vi "Versioned Load.vi"(5 "path":path) -> (1 "Overall":cluster{"Time (s)":dbl, "Distance (ft)":dbl}, 3 "Points out":cluster{"x":dbl, "y":dbl, "th":dbl}[](array[cluster]), 4 "Commands out":cluster{"Time (s)":dbl, T8, bool}[](array[cluster]), 6 "Zero V":bool, 8 "Reversals":T10, 10 "Trajectory Data":T1, 12 "Trajectory Meta":cluster{"Drive Type":T3, "Path Type":T4}, 14 "Fields":T7 {"Overrides"."Angle Override" step=5.0; "Overrides"."Velocity Override" step=5.0; "Overrides"."Angular Override" step=5.0; "Angular Limits"."Jerk (deg/s^3)" min=0.0 step=1.0; "Angular Limits"."Accel (deg/s^2)" min=0.0; "Angular Limits"."Velocity (deg/s)" min=0.0}, 15 "Auto Align":bool)   [LabVIEW 2025]
uses:
  Types/Single Cmd Info.ctl
  <vilib>/picture/picture.llb/imagedata.ctl
  Types/Overrides.ctl
  Types/Angluar Limits.ctl
  Types/Drive Type.ctl
  Types/Path Type.ctl
  Types/Trajectory Data.ctl
  Types/Segment Type.ctl
  Types/Availible Command systems for auto.ctl
  Types/Limits.ctl
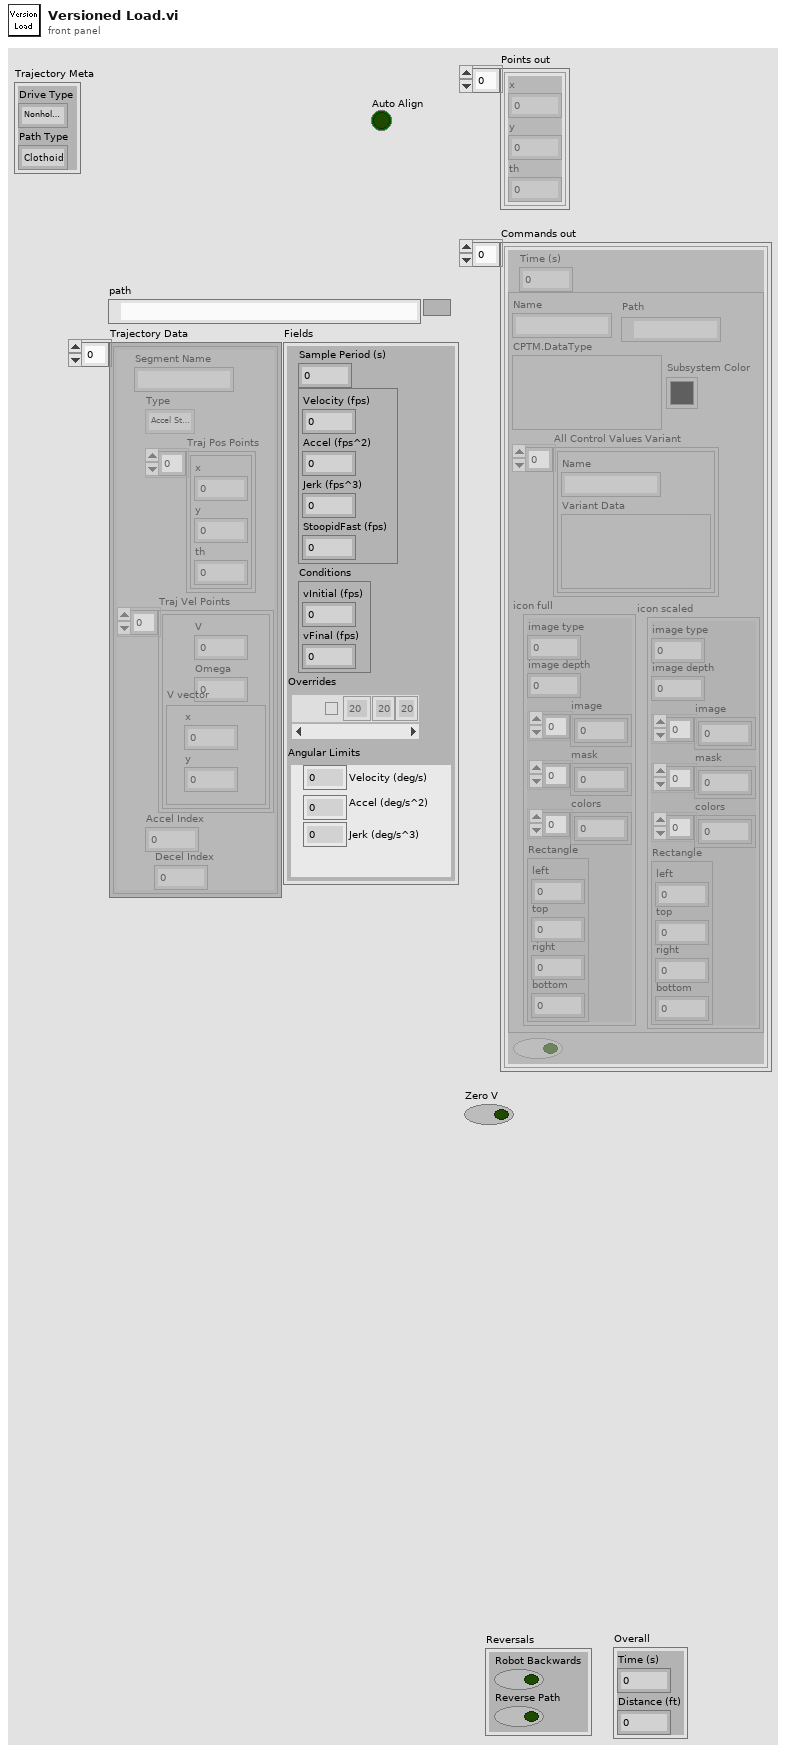
[diagram p1: front panel]
types:
  T1 = typedef "Trajectory Data.ctl" = cluster{"Segment Name":string, "Type":T2, "Traj Pos Points":cluster{"x":dbl, "y":dbl, "th":dbl}[], "Traj Vel Points":cluster{"V":dbl, "Omega":dbl, "V vector":cluster{"y":dbl, "x":dbl}}[], "Accel Index":i32, "Decel Index":i32}[]
  T2 = typedef "Segment Type.ctl" = enum16{"Accel Straight", "Const Straight", "Blend", "Circle", "Bezier"}
  T3 = typedef "Drive Type.ctl" = enum16{"Nonholonomic", "Holonomic"}
  T4 = typedef "Path Type.ctl" = enum16{"Clothoid", "Bezier"}
  T5 = typedef "Overrides.ctl" = cluster{"Count":string, "Angular Override":dbl, "Enabled?":bool, "Velocity Override":dbl, "Angle Override":dbl}[]
  T6 = typedef "Angluar Limits.ctl" = cluster{"Velocity (deg/s)":dbl, "Accel (deg/s^2)":dbl, "Jerk (deg/s^3)":dbl}
  T7 = cluster{"Sample Period (s)":dbl, cluster{"Velocity (fps)":dbl, "Accel (fps^2)":dbl, "Jerk (fps^3)":dbl, "StoopidFast (fps)":dbl}, "Conditions":cluster{"vInitial (fps)":dbl, "vFinal (fps)":dbl}, "Overrides":T5, "Angular Limits":T6}
  T8 = typedef "Single Cmd Info.ctl" = cluster{"Name":string, "CPTM.DataType":variant, "All Control Values Variant":cluster{"Name":string, "Variant Data":variant}[], "icon full":T9, "icon scaled":T9, "Path":path, "Subsystem Color":u32}
  T9 = typedef "imagedata.ctl" = cluster{"image type":i32, "image depth":i32, "image":u8[], "mask":u8[], "colors":u32[], "Rectangle":cluster{"left":i16, "top":i16, "right":i16, "bottom":i16}}
  T10 = cluster{"Robot Backwards":bool, "Reverse Path":bool}
  T11 = cluster{"Segment Name":string, "Type":T2, "Traj Pos Points":cluster{"x":dbl, "y":dbl, "th":dbl}[], "Traj Vel Points":cluster{"V":dbl, "Omega":dbl}[], "Accel Index":i32, "Decel Index":i32}[]
  T12 = cluster{"Sample Period (s)":dbl, "Limits 2":cluster{"Velocity (fps)":dbl, "Acceleration (fps^2)":dbl, "Jerk (fps^3)":dbl}, "Conditions":cluster{"vInitial (fps)":dbl, "vFinal (fps)":dbl}, " Acceleration Overrides":cluster{"Angular \nAccelerations":dbl[], "Accel Override Bools":bool[]}}
  T13 = cluster{"Velocity":dbl, "Sample Time":dbl, "Accel":dbl}
  T14 = cluster{"Sample Period (s)":dbl, "Limits":cluster{"Velocity (fps)":dbl, "Acceleration (fps^2)":dbl, "Jerk (fps^3)":dbl}, "Conditions":cluster{"vInitial (fps)":dbl, "vFinal (fps)":dbl}}
  T15 = cluster{"Sample Period (s)":dbl, "Limits":cluster{"Velocity (fps)":dbl, "Acceleration (fps^2)":dbl, "Jerk (fps^3)":dbl}, "Conditions":cluster{"vInitial (fps)":dbl, "vFinal (fps)":dbl}, "Min Rads":dbl[]}
  T16 = typedef "Availible Command systems for auto.ctl" = u16
  T17 = cluster{"Time into Path":dbl, "System":T16, "Item Selected?":bool, "System Selection":T16}[]
  T18 = cluster{"Sample Period (s)":dbl, "Limits 2":cluster{"Velocity (fps)":dbl, "Acceleration (fps^2)":dbl, "Jerk (fps^3)":dbl, "Stoopid Fast":dbl}, "Conditions":cluster{"vInitial (fps)":dbl, "vFinal (fps)":dbl}, " Acceleration Overrides":cluster{"Angular \nAccelerations":dbl[], "Accel Override Bools":bool[]}}
  T19 = cluster{"Sample Period (s)":dbl, "Limits":cluster{"Velocity (fps)":dbl, "Accel (fps^2)":dbl, "Turn Accel (fps^2)":dbl, "Jerk (fps^3)":dbl}, "Conditions":cluster{"vInitial (fps)":dbl, "vFinal (fps)":dbl}, cluster{dbl[], bool[]}}
  T20 = cluster{"Reverse Path":bool, "Robot Backwards":bool}
  T21 = typedef "Limits.ctl" = cluster{"Velocity (fps)":dbl, "Accel (fps^2)":dbl, "Jerk (fps^3)":dbl, "StoopidFast (fps)":dbl}
  T22 = cluster{"Sample Period (s)":dbl, "Limits":T21, "Conditions":cluster{"vInitial (fps)":dbl, "vFinal (fps)":dbl}, "Overrides":T5, "Angular Limits":T6}
  T23 = cluster{"Velocity":dbl, "Accel":dbl, "Accel":dbl, "Velocity":dbl}
  T24 = cluster{"Velocity (fps)":dbl, "Acceleration (fps^2)":dbl, "Jerk (fps^3)":dbl}
  T25 = cluster{"vInitial (fps)":dbl, "vFinal (fps)":dbl}
  T26 = cluster{"Velocity (fps)":dbl, "Acceleration (fps^2)":dbl, "Jerk (fps^3)":dbl, "Velocity (fps)":dbl}
  T27 = cluster{string, "Angular Multiplier":dbl, bool, "Velocity (fps)":dbl, "Velocity (fps)":dbl}
  T28 = cluster{"Angular \nAccelerations":dbl[], "Accel Override Bools":bool[]}
  T29 = cluster{"Velocity (fps)":dbl, "Acceleration (fps^2)":dbl, "Jerk (fps^3)":dbl, "Stoopid Fast":dbl}
  T30 = cluster{"Velocity (fps)":dbl, "Accel (fps^2)":dbl, "Turn Accel (fps^2)":dbl, "Jerk (fps^3)":dbl}
  T31 = cluster{"Velocity (fps)":dbl, "Accel (fps^2)":dbl, "Jerk (fps^3)":dbl, "StoopidFast (fps)":dbl}
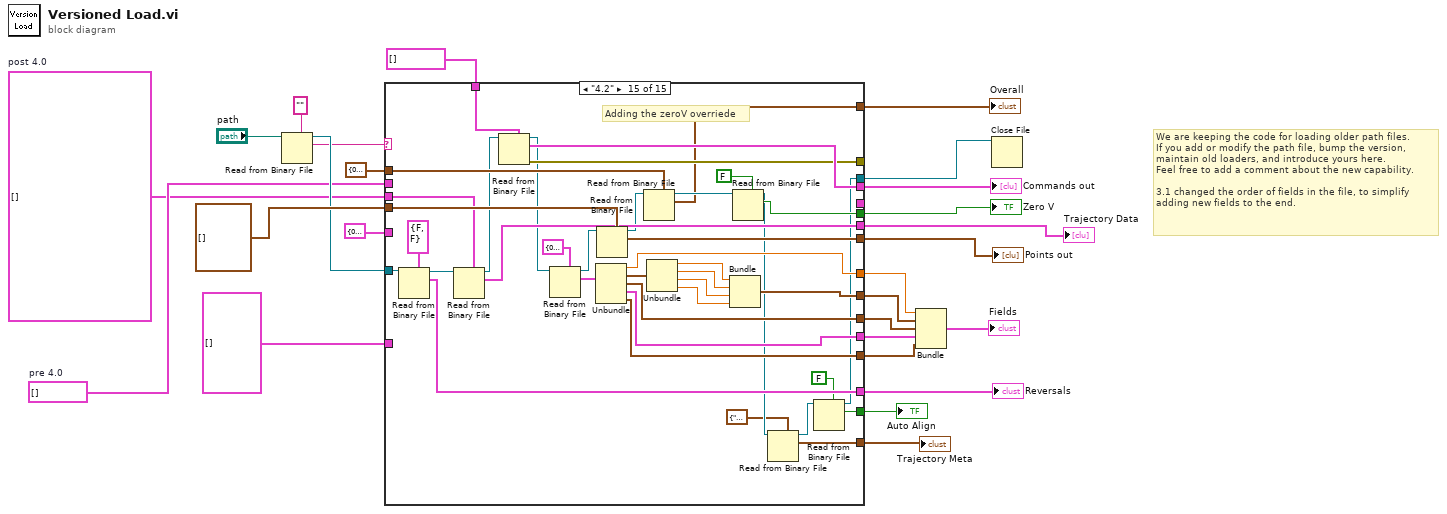
[diagram p0: block diagram]
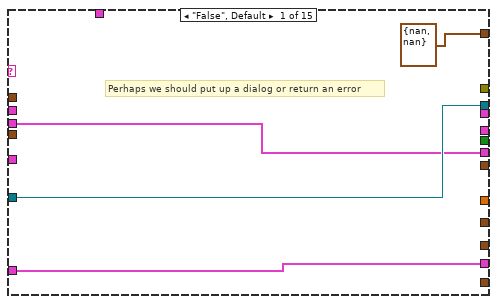
[diagram p2: hidden frame]
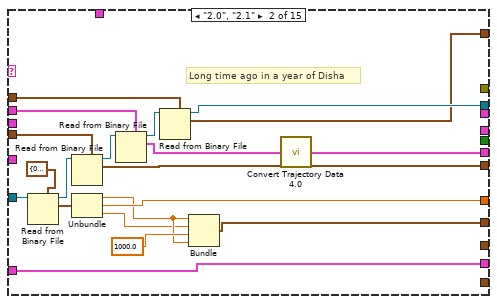
[diagram p3: hidden frame]
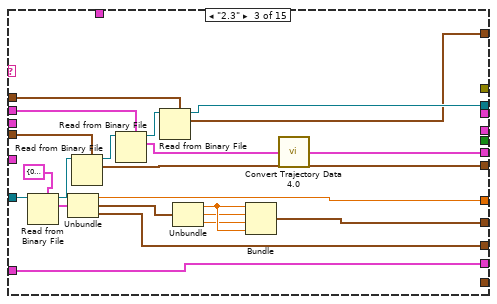
[diagram p4: hidden frame]
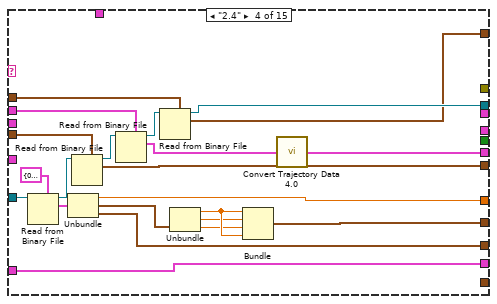
[diagram p5: hidden frame]
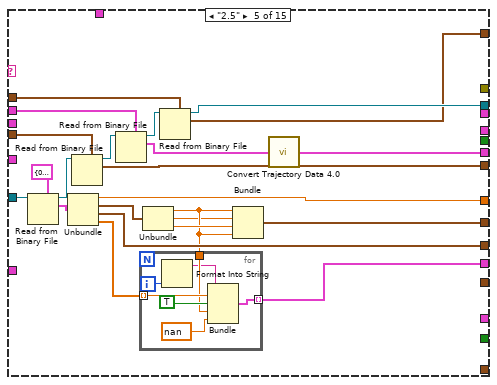
[diagram p6: hidden frame]
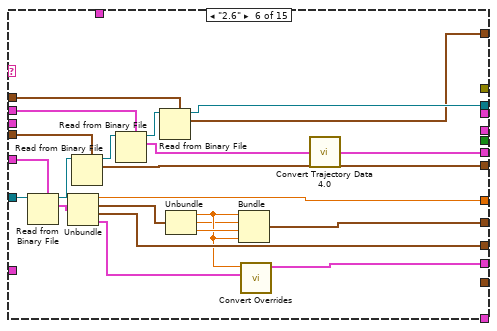
[diagram p7: hidden frame]
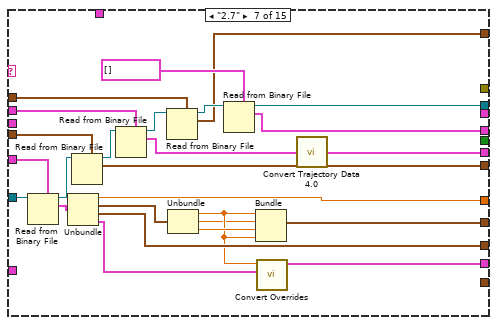
[diagram p8: hidden frame]
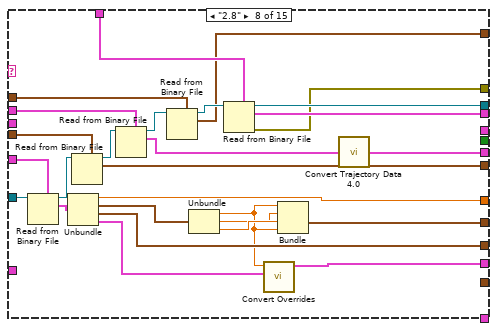
[diagram p9: hidden frame]
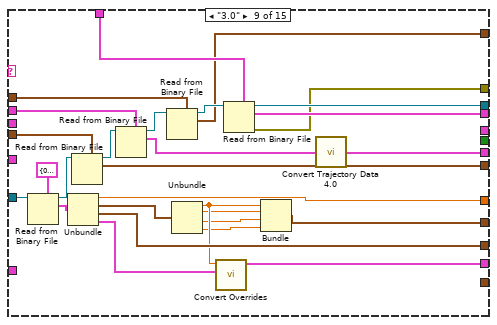
[diagram p10: hidden frame]
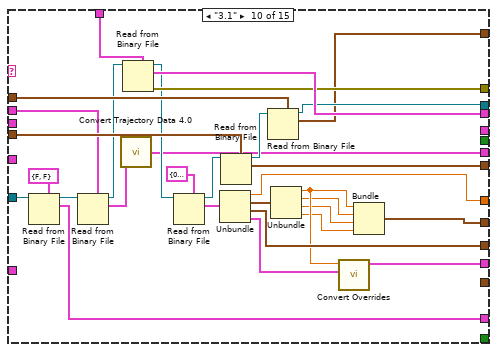
[diagram p11: hidden frame]
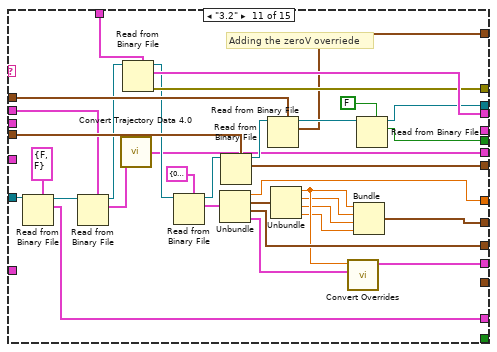
[diagram p12: hidden frame]
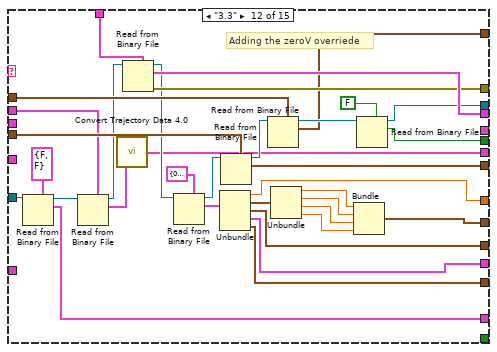
[diagram p13: hidden frame]
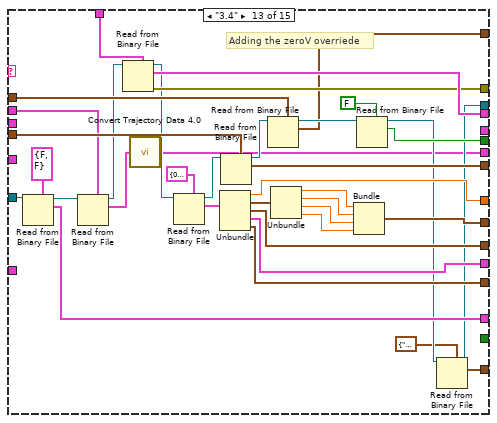
[diagram p14: hidden frame]
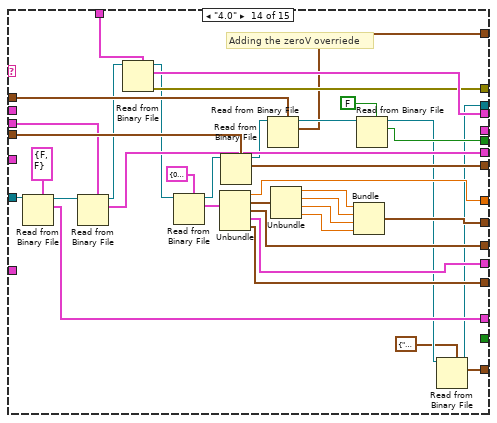
[diagram p15: hidden frame]
diagram:
  w4 = T11 []  # pre 4.0
  w3 = T1 []  # post 4.0
  # "We are keeping the code for loading older path files.\nIf you add or modify the path file, bump the version,\nmaintain old loaders, and introduce yours here.\nFeel free to add a comment about the new capability.\n\n3.1 changed the order of fields in the file, to simplify\nadding new fields to the end."
  n1 = Read from Binary File(5:"" ("String"), 11:"path") -> (2:w10:string, 3:w11:refnum<file>)  [unwired: 4 in, 2 out]
  n2 = case shown="\"4.2\"" w10 {
    tunnel: w11 -> [w30 w49 w71 w93 w116 w146 w172 w199 w227 w248 w282 w316 w353 w390 w429]
    tunnel: cluster{"x":dbl, "y":dbl, "th":dbl}[] [] ("Points in") -> [_ w47 w69 w91 w114 w144 w170 w197 w225 w257 w291 w325 w362 w398 w437]
    tunnel: [_ w46 w68 w90 w113 w143 w169 w196 w224 w256 w290 w324 w361 w397 w436] -> w16
    tunnel: w4 -> [_ w45 w67 w89 w112 w142 w168 w195 w223 w255 w289 w323 w360 _ _]
    tunnel: cluster{"Time (s)":dbl, "Distance (ft)":dbl} {"Time (s)"=0.0, "Distance (ft)"=0.0} ("Cluster 4") -> [_ w43 w65 w87 w110 w140 w166 w193 w221 w254 w288 w322 w359 w396 w435]
    tunnel: [w30 w41 w63 w85 w108 w138 w160 w187 w215 w244 w264 w301 w330 w367 w403] -> w13
    tunnel: [_ w39 w62 w84 w107 w137 w164 w191 w219 w231 w266 w303 w340 w377 w416] -> w23
    tunnel: [_ w35 w56 w77 w101 w132 w154 w182 w203 w236 w271 w308 w345 w382 w421] -> w24
    tunnel: [_ _ w61 w83 w106 w136 w163 w190 w218 w253 w287 w321 w358 w395 w434] -> w25
    tunnel: [w29 w34 w55 w76 w100 w130 w151 w179 w209 w240 w275 w296 w334 w371 w410] -> w26
    tunnel: [w27 w31 w51 w73 w95 w125 w148 w174 w201 w229 w260 w294 w328 w394 w433] -> w2
    tunnel: [_ _ _ _ _ _ w159 _ _ _ _ _ _ _ _] -> _
    tunnel: cluster{"Time (s)":dbl, T8, bool}[] [] ("Commands in") -> [_ _ _ _ _ _ _ w186 w214 w251 w285 w319 w356 w393 w432]
    tunnel: [_ _ _ _ _ _ _ w185 w213 w250 w284 w318 w355 w392 w431] -> w18
    tunnel: [_ _ _ _ _ _ _ w184 w212 w249 w283 w317 w354 w391 w430] -> _
    tunnel: T12 {"Sample Period (s)"=0.0, "Limits 2"={"Velocity (fps)"=0.0, "Acceleration (fps^2)"=0.0, "Jerk (fps^3)"=0.0}, "Conditions"={"vInitial (fps)"=0.0, "vFinal (fps)"=0.0}, " Acceleration Overrides"={"Angular \nAccelerations"=[], "Accel Override Bools"=[]}} ("Cluster") -> [_ _ _ _ _ w134 w157 w180 _ _ _ _ _ _ _]
    tunnel: [_ _ _ _ _ _ _ _ _ w239 w274 w310 w347 w384 w423] -> w20
    tunnel: T5 [] ("Overrides") -> [w29 w34 w55 w76 _ _ _ _ _ _ _ _ _ _ _]
    tunnel: [_ _ _ _ _ _ _ _ _ _ w262 w299 w337 w374 w413] -> w21
    tunnel: [cluster{"Time (s)":dbl, "Distance (ft)":dbl} {"Time (s)"=nan, "Distance (ft)"=nan} ("Cluster 4") w32 w52 w74 w96 w126 w149 w175 w202 w230 w261 w298 w336 w373 w412] -> w8
    tunnel: [_ _ _ _ _ _ _ _ _ _ _ w295 w333 w370 w409] -> w6
    tunnel: [_ _ _ _ _ _ _ _ _ _ _ _ w329 w366 w406] -> w5
    tunnel: w3 -> [w27 _ _ _ _ _ _ _ _ _ _ _ _ w365 w405]
    tunnel: [_ _ _ _ _ _ _ _ _ _ _ _ _ _ w401] -> w1
    frame "False", Default {
      # "Perhaps we should put up a dialog or return an error"
    }
    frame "2.0", "2.1" {
      # "Long time ago in a year of Disha"
      n3 = Read from Binary File(5:T13 {"Velocity"=0.0, "Sample Time"=0.0, "Accel"=0.0}, 11:w49) -> (2:w50:T13, 3:w48:refnum<file>)  [unwired: 4 in, 2 out]
      n4 = Read from Binary File(5:w47, 11:w48) -> (2:w46:cluster{"x":dbl, "y":dbl, "th":dbl}[], 3:w44:refnum<file>)  [unwired: 4 in, 2 out]
      n5 = Unbundle(w50) -> ("Velocity"=w36:dbl, "Sample Time"=w39:dbl, "Accel"=w33:dbl)
      n6 = Read from Binary File(5:w45, 11:w44) -> (2:w37:T11, 3:w42:refnum<file>)  [unwired: 4 in, 2 out]
      n7 = Read from Binary File(5:w43, 11:w42) -> (2:w32:cluster{"Time (s)":dbl, "Distance (ft)":dbl}, 3:w41:refnum<file>)  [unwired: 4 in, 2 out]
      n8 = Bundle("Velocity"=w36, "Accel"=w33, "Accel"=1000.0, "Velocity"=w36) -> (w35:T23)  [unwired: 1 in]
      n9 = call "Convert Trajectory Data 4.0.vi"("pre 4.0"=w37) -> ("post 4.0"=w31:T1)
    }
    frame "2.3" {
      n10 = Read from Binary File(5:T14 {"Sample Period (s)"=0.0, "Limits"={"Velocity (fps)"=0.0, "Acceleration (fps^2)"=0.0, "Jerk (fps^3)"=0.0}, "Conditions"={"vInitial (fps)"=0.0, "vFinal (fps)"=0.0}}, 11:w71) -> (2:w72:T14, 3:w70:refnum<file>)  [unwired: 4 in, 2 out]
      n11 = Unbundle(w72) -> ("Sample Period (s)"=w62:dbl, "Limits"=w53:T24, "Conditions"=w61:T25)
      n12 = Read from Binary File(5:w69, 11:w70) -> (2:w68:cluster{"x":dbl, "y":dbl, "th":dbl}[], 3:w66:refnum<file>)  [unwired: 4 in, 2 out]
      n13 = Read from Binary File(5:w67, 11:w66) -> (2:w59:T11, 3:w64:refnum<file>)  [unwired: 4 in, 2 out]
      n14 = Read from Binary File(5:w65, 11:w64) -> (2:w52:cluster{"Time (s)":dbl, "Distance (ft)":dbl}, 3:w63:refnum<file>)  [unwired: 4 in, 2 out]
      n15 = Unbundle(w53) -> ("Velocity (fps)"=w58:dbl, "Acceleration (fps^2)"=w54:dbl, "Jerk (fps^3)"=w57:dbl)
      n16 = Bundle("Velocity (fps)"=w58, "Acceleration (fps^2)"=w54, "Jerk (fps^3)"=w57, "Velocity (fps)"=w58) -> (w56:T26)  [unwired: 1 in]
      n17 = call "Convert Trajectory Data 4.0.vi"("pre 4.0"=w59) -> ("post 4.0"=w51:T1)
    }
    frame "2.4" {
      n18 = Read from Binary File(5:T14 {"Sample Period (s)"=0.0, "Limits"={"Velocity (fps)"=0.0, "Acceleration (fps^2)"=0.0, "Jerk (fps^3)"=0.0}, "Conditions"={"vInitial (fps)"=0.0, "vFinal (fps)"=0.0}}, 11:w93) -> (2:w94:T14, 3:w92:refnum<file>)  [unwired: 4 in, 2 out]
      n19 = Unbundle(w94) -> ("Sample Period (s)"=w84:dbl, "Limits"=w78:T24, "Conditions"=w83:T25)
      n20 = Read from Binary File(5:w91, 11:w92) -> (2:w90:cluster{"x":dbl, "y":dbl, "th":dbl}[], 3:w88:refnum<file>)  [unwired: 4 in, 2 out]
      n21 = Read from Binary File(5:w89, 11:w88) -> (2:w81:T11, 3:w86:refnum<file>)  [unwired: 4 in, 2 out]
      n22 = Read from Binary File(5:w87, 11:w86) -> (2:w74:cluster{"Time (s)":dbl, "Distance (ft)":dbl}, 3:w85:refnum<file>)  [unwired: 4 in, 2 out]
      n23 = Unbundle(w78) -> ("Velocity (fps)"=w80:dbl, "Acceleration (fps^2)"=w75:dbl, "Jerk (fps^3)"=w79:dbl)
      n24 = Bundle("Velocity (fps)"=w80, "Acceleration (fps^2)"=w75, "Jerk (fps^3)"=w79, "Velocity (fps)"=w80) -> (w77:T26)  [unwired: 1 in]
      n25 = call "Convert Trajectory Data 4.0.vi"("pre 4.0"=w81) -> ("post 4.0"=w73:T1)
    }
    frame "2.5" {
      n26 = Read from Binary File(5:T15 {"Sample Period (s)"=0.0, "Limits"={"Velocity (fps)"=0.0, "Acceleration (fps^2)"=0.0, "Jerk (fps^3)"=0.0}, "Conditions"={"vInitial (fps)"=0.0, "vFinal (fps)"=0.0}, "Min Rads"=[20.0, 20.0, 20.0, 20.0, 20.0]}, 11:w116) -> (2:w117:T15, 3:w115:refnum<file>)  [unwired: 4 in, 2 out]
      n27 = Unbundle(w117) -> ("Sample Period (s)"=w107:dbl, "Limits"=w102:T24, "Conditions"=w106:T25, "Min Rads"=w99:dbl[])
      n28 = Read from Binary File(5:w114, 11:w115) -> (2:w113:cluster{"x":dbl, "y":dbl, "th":dbl}[], 3:w111:refnum<file>)  [unwired: 4 in, 2 out]
      n29 = Read from Binary File(5:w112, 11:w111) -> (2:w104:T11, 3:w109:refnum<file>)  [unwired: 4 in, 2 out]
      n30 = Unbundle(w102) -> ("Velocity (fps)"=w98:dbl, "Acceleration (fps^2)"=w97:dbl, "Jerk (fps^3)"=w103:dbl)
      n31 = for {
        tunnel: [w123] -> w100 mode=indexing
        tunnel: w99 -> [w122] mode=indexing
        tunnel: w98 -> [w121]
        i -> [w120]
        n32 = Format Into String(w120) -> (resulting string=w119:string)  [unwired: 3 in, 1 out]
        n33 = Bundle(w119, "Angular Multiplier"=w122, TRUE, "Velocity (fps)"=w121, "Velocity (fps)"=nan) -> (w123:T27)  [unwired: 1 in]
      }
      n34 = Read from Binary File(5:w110, 11:w109) -> (2:w96:cluster{"Time (s)":dbl, "Distance (ft)":dbl}, 3:w108:refnum<file>)  [unwired: 4 in, 2 out]
      n35 = Bundle("Velocity (fps)"=w98, "Acceleration (fps^2)"=w97, "Jerk (fps^3)"=w103, "Velocity (fps)"=w98) -> (w101:T26)  [unwired: 1 in]
      n36 = call "Convert Trajectory Data 4.0.vi"("pre 4.0"=w104) -> ("post 4.0"=w95:T1)
    }
    frame "2.6" {
      n37 = Read from Binary File(5:w134, 11:w146) -> (2:w147:T12, 3:w145:refnum<file>)  [unwired: 4 in, 2 out]
      n38 = Unbundle(w147) -> ("Sample Period (s)"=w137:dbl, "Limits 2"=w131:T24, "Conditions"=w136:T25, "Acceleration Overrides"=w128:T28)
      n39 = Read from Binary File(5:w144, 11:w145) -> (2:w143:cluster{"x":dbl, "y":dbl, "th":dbl}[], 3:w141:refnum<file>)  [unwired: 4 in, 2 out]
      n40 = Read from Binary File(5:w142, 11:w141) -> (2:w135:T11, 3:w139:refnum<file>)  [unwired: 4 in, 2 out]
      n41 = Read from Binary File(5:w140, 11:w139) -> (2:w126:cluster{"Time (s)":dbl, "Distance (ft)":dbl}, 3:w138:refnum<file>)  [unwired: 4 in, 2 out]
      n42 = Unbundle(w131) -> ("Velocity (fps)"=w129:dbl, "Acceleration (fps^2)"=w127:dbl, "Jerk (fps^3)"=w133:dbl)
      n43 = Bundle("Velocity (fps)"=w129, "Acceleration (fps^2)"=w127, "Jerk (fps^3)"=w133, "Velocity (fps)"=w129) -> (w132:T26)  [unwired: 1 in]
      n44 = call "Convert Overrides.vi"("Cluster"=w128, "Velocity (fps)"=w129) -> ("Overrides"=w130:T5)  [unwired: 9 in]
      n45 = call "Convert Trajectory Data 4.0.vi"("pre 4.0"=w135) -> ("post 4.0"=w125:T1)
    }
    frame "2.7" {
      n46 = Read from Binary File(5:w157, 11:w172) -> (2:w173:T12, 3:w171:refnum<file>)  [unwired: 4 in, 2 out]
      n47 = Unbundle(w173) -> ("Sample Period (s)"=w164:dbl, "Limits 2"=w155:T24, "Conditions"=w163:T25, "Acceleration Overrides"=w152:T28)
      n48 = Read from Binary File(5:w170, 11:w171) -> (2:w169:cluster{"x":dbl, "y":dbl, "th":dbl}[], 3:w167:refnum<file>)  [unwired: 4 in, 2 out]
      n49 = Read from Binary File(5:w168, 11:w167) -> (2:w162:T11, 3:w165:refnum<file>)  [unwired: 4 in, 2 out]
      n50 = Read from Binary File(5:w166, 11:w165) -> (2:w149:cluster{"Time (s)":dbl, "Distance (ft)":dbl}, 3:w161:refnum<file>)  [unwired: 4 in, 2 out]
      n51 = Unbundle(w155) -> ("Velocity (fps)"=w153:dbl, "Acceleration (fps^2)"=w150:dbl, "Jerk (fps^3)"=w156:dbl)
      n52 = Read from Binary File(5:T17 [] ("Commands"), 11:w161) -> (2:w159:T17, 3:w160:refnum<file>)  [unwired: 4 in, 2 out]
      n53 = Bundle("Velocity (fps)"=w153, "Acceleration (fps^2)"=w150, "Jerk (fps^3)"=w156, "Velocity (fps)"=w153) -> (w154:T26)  [unwired: 1 in]
      n54 = call "Convert Overrides.vi"("Cluster"=w152, "Velocity (fps)"=w153) -> ("Overrides"=w151:T5)  [unwired: 9 in]
      n55 = call "Convert Trajectory Data 4.0.vi"("pre 4.0"=w162) -> ("post 4.0"=w148:T1)
    }
    frame "2.8" {
      n56 = Read from Binary File(5:w180, 11:w199) -> (2:w200:T12, 3:w198:refnum<file>)  [unwired: 4 in, 2 out]
      n57 = Unbundle(w200) -> ("Sample Period (s)"=w191:dbl, "Limits 2"=w183:T24, "Conditions"=w190:T25, "Acceleration Overrides"=w177:T28)
      n58 = Read from Binary File(5:w197, 11:w198) -> (2:w196:cluster{"x":dbl, "y":dbl, "th":dbl}[], 3:w194:refnum<file>)  [unwired: 4 in, 2 out]
      n59 = Read from Binary File(5:w195, 11:w194) -> (2:w189:T11, 3:w192:refnum<file>)  [unwired: 4 in, 2 out]
      n60 = Read from Binary File(5:w193, 11:w192) -> (2:w175:cluster{"Time (s)":dbl, "Distance (ft)":dbl}, 3:w188:refnum<file>)  [unwired: 4 in, 2 out]
      n61 = Unbundle(w183) -> ("Velocity (fps)"=w178:dbl, "Acceleration (fps^2)"=w176:dbl, "Jerk (fps^3)"=w181:dbl)
      n62 = Read from Binary File(5:w186, 11:w188) -> (0:w184:errorcluster, 2:w185:cluster{"Time (s)":dbl, T8, bool}[], 3:w187:refnum<file>)  [unwired: 4 in, 1 out]
      n63 = call "Convert Overrides.vi"("Cluster"=w177, "Velocity (fps)"=w178) -> ("Overrides"=w179:T5)  [unwired: 9 in]
      n64 = Bundle("Velocity (fps)"=w178, "Acceleration (fps^2)"=w176, "Jerk (fps^3)"=w181, "Velocity (fps)"=w178) -> (w182:T26)  [unwired: 1 in]
      n65 = call "Convert Trajectory Data 4.0.vi"("pre 4.0"=w189) -> ("post 4.0"=w174:T1)
    }
    frame "3.0" {
      n66 = Read from Binary File(5:T18 {"Sample Period (s)"=0.0, "Limits 2"={"Velocity (fps)"=0.0, "Acceleration (fps^2)"=0.0, "Jerk (fps^3)"=0.0, "Stoopid Fast"=0.0}, "Conditions"={"vInitial (fps)"=0.0, "vFinal (fps)"=0.0}, " Acceleration Overrides"={"Angular \nAccelerations"=[], "Accel Override Bools"=[]}} ("Cluster"), 11:w227) -> (2:w228:T18, 3:w226:refnum<file>)  [unwired: 4 in, 2 out]
      n67 = Unbundle(w228) -> ("Sample Period (s)"=w219:dbl, "Limits 2"=w204:T29, "Conditions"=w218:T25, "Acceleration Overrides"=w210:T28)
      n68 = Read from Binary File(5:w225, 11:w226) -> (2:w224:cluster{"x":dbl, "y":dbl, "th":dbl}[], 3:w222:refnum<file>)  [unwired: 4 in, 2 out]
      n69 = Read from Binary File(5:w223, 11:w222) -> (2:w217:T11, 3:w220:refnum<file>)  [unwired: 4 in, 2 out]
      n70 = Read from Binary File(5:w221, 11:w220) -> (2:w202:cluster{"Time (s)":dbl, "Distance (ft)":dbl}, 3:w216:refnum<file>)  [unwired: 4 in, 2 out]
      n71 = Unbundle(w204) -> ("Velocity (fps)"=w208:dbl, "Acceleration (fps^2)"=w207:dbl, "Jerk (fps^3)"=w206:dbl, "Stoopid Fast"=w205:dbl)
      n72 = call "Convert Overrides.vi"("Cluster"=w210, "Velocity (fps)"=w208) -> ("Overrides"=w209:T5)  [unwired: 9 in]
      n73 = Read from Binary File(5:w214, 11:w216) -> (0:w212:errorcluster, 2:w213:cluster{"Time (s)":dbl, T8, bool}[], 3:w215:refnum<file>)  [unwired: 4 in, 1 out]
      n74 = Bundle("Velocity (fps)"=w208, "Acceleration (fps^2)"=w207, "Jerk (fps^3)"=w206, "Stoopid Fast"=w205) -> (w203:T29)  [unwired: 1 in]
      n75 = call "Convert Trajectory Data 4.0.vi"("pre 4.0"=w217) -> ("post 4.0"=w201:T1)
    }
    frame "3.1" {
      n76 = Read from Binary File(5:T20 {"Reverse Path"=FALSE, "Robot Backwards"=FALSE} ("Cluster"), 11:w248) -> (2:w239:T20, 3:w245:refnum<file>)  [unwired: 4 in, 2 out]
      n77 = Read from Binary File(5:w255, 11:w245) -> (2:w252:T11, 3:w243:refnum<file>)  [unwired: 4 in, 2 out]
      n78 = call "Convert Trajectory Data 4.0.vi"("pre 4.0"=w252) -> ("post 4.0"=w229:T1)
      n79 = Read from Binary File(5:w251, 11:w243) -> (0:w249:errorcluster, 2:w250:cluster{"Time (s)":dbl, T8, bool}[], 3:w242:refnum<file>)  [unwired: 4 in, 1 out]
      n80 = Read from Binary File(5:T19 {"Sample Period (s)"=0.0, "Limits"={"Velocity (fps)"=0.0, "Accel (fps^2)"=0.0, "Turn Accel (fps^2)"=15.0, "Jerk (fps^3)"=0.0}, "Conditions"={"vInitial (fps)"=0.0, "vFinal (fps)"=0.0}, {[], []}} ("Cluster 2"), 11:w242) -> (2:w259:T19, 3:w258:refnum<file>)  [unwired: 4 in, 2 out]
      n81 = Unbundle(w259) -> ("Sample Period (s)"=w231:dbl, "Limits"=w238:T30, "Conditions"=w253:T25, w241:cluster{dbl[], bool[]})
      n82 = Read from Binary File(5:w257, 11:w258) -> (2:w256:cluster{"x":dbl, "y":dbl, "th":dbl}[], 3:w246:refnum<file>)  [unwired: 4 in, 2 out]
      n83 = Read from Binary File(5:w254, 11:w246) -> (2:w230:cluster{"Time (s)":dbl, "Distance (ft)":dbl}, 3:w244:refnum<file>)  [unwired: 4 in, 2 out]
      n84 = Unbundle(w238) -> ("Velocity (fps)"=w235:dbl, "Accel (fps^2)"=w234:dbl, "Turn Accel (fps^2)"=w233:dbl, "Jerk (fps^3)"=w232:dbl)
      n85 = call "Convert Overrides.vi"("Cluster"=w241, "Velocity (fps)"=w235) -> ("Overrides"=w240:T5)  [unwired: 9 in]
      n86 = Bundle("Velocity (fps)"=w235, "Accel (fps^2)"=w234, "Turn Accel (fps^2)"=w233, "Jerk (fps^3)"=w232) -> (w236:T30)  [unwired: 1 in]
    }
    frame "3.2" {
      # "Adding the zeroV overriede"
      n87 = Read from Binary File(5:T10 {"Robot Backwards"=FALSE, "Reverse Path"=FALSE} ("Cluster"), 11:w282) -> (2:w274:T10, 3:w279:refnum<file>)  [unwired: 4 in, 2 out]
      n88 = Read from Binary File(5:w289, 11:w279) -> (2:w286:T11, 3:w278:refnum<file>)  [unwired: 4 in, 2 out]
      n89 = call "Convert Trajectory Data 4.0.vi"("pre 4.0"=w286) -> ("post 4.0"=w260:T1)
      n90 = Read from Binary File(5:w285, 11:w278) -> (0:w283:errorcluster, 2:w284:cluster{"Time (s)":dbl, T8, bool}[], 3:w277:refnum<file>)  [unwired: 4 in, 1 out]
      n91 = Read from Binary File(5:T19 {"Sample Period (s)"=0.0, "Limits"={"Velocity (fps)"=0.0, "Accel (fps^2)"=0.0, "Turn Accel (fps^2)"=15.0, "Jerk (fps^3)"=0.0}, "Conditions"={"vInitial (fps)"=0.0, "vFinal (fps)"=0.0}, {[], []}} ("Cluster 2"), 11:w277) -> (2:w293:T19, 3:w292:refnum<file>)  [unwired: 4 in, 2 out]
      n92 = Unbundle(w293) -> ("Sample Period (s)"=w266:dbl, "Limits"=w273:T30, "Conditions"=w287:T25, w276:cluster{dbl[], bool[]})
      n93 = Read from Binary File(5:w291, 11:w292) -> (2:w290:cluster{"x":dbl, "y":dbl, "th":dbl}[], 3:w280:refnum<file>)  [unwired: 4 in, 2 out]
      n94 = Read from Binary File(5:w288, 11:w280) -> (2:w261:cluster{"Time (s)":dbl, "Distance (ft)":dbl}, 3:w265:refnum<file>)  [unwired: 4 in, 2 out]
      n95 = Unbundle(w273) -> ("Velocity (fps)"=w270:dbl, "Accel (fps^2)"=w269:dbl, "Turn Accel (fps^2)"=w268:dbl, "Jerk (fps^3)"=w267:dbl)
      n96 = call "Convert Overrides.vi"("Cluster"=w276, "Velocity (fps)"=w270) -> ("Overrides"=w275:T5)  [unwired: 9 in]
      n97 = Bundle("Velocity (fps)"=w270, "Accel (fps^2)"=w269, "Turn Accel (fps^2)"=w268, "Jerk (fps^3)"=w267) -> (w271:T30)  [unwired: 1 in]
      n98 = Read from Binary File(5:FALSE, 11:w265) -> (2:w262:bool, 3:w264:refnum<file>)  [unwired: 4 in, 2 out]
    }
    frame "3.3" {
      # "Adding the zeroV overriede"
      n99 = Read from Binary File(5:T10 {"Robot Backwards"=FALSE, "Reverse Path"=FALSE} ("Cluster"), 11:w316) -> (2:w310:T10, 3:w313:refnum<file>)  [unwired: 4 in, 2 out]
      n100 = Read from Binary File(5:w323, 11:w313) -> (2:w320:T11, 3:w312:refnum<file>)  [unwired: 4 in, 2 out]
      n101 = call "Convert Trajectory Data 4.0.vi"("pre 4.0"=w320) -> ("post 4.0"=w294:T1)
      n102 = Read from Binary File(5:w319, 11:w312) -> (0:w317:errorcluster, 2:w318:cluster{"Time (s)":dbl, T8, bool}[], 3:w311:refnum<file>)  [unwired: 4 in, 1 out]
      n103 = Read from Binary File(5:T22 {"Sample Period (s)"=0.0, "Limits"={"Velocity (fps)"=0.0, "Accel (fps^2)"=0.0, "Jerk (fps^3)"=0.0, "StoopidFast (fps)"=0.0}, "Conditions"={"vInitial (fps)"=0.0, "vFinal (fps)"=0.0}, "Overrides"=[], "Angular Limits"={"Velocity (deg/s)"=0.0, "Accel (deg/s^2)"=0.0, "Jerk (deg/s^3)"=0.0}} ("output cluster"), 11:w311) -> (2:w327:T22, 3:w326:refnum<file>)  [unwired: 4 in, 2 out]
      n104 = Unbundle(w327) -> ("Sample Period (s)"=w303:dbl, "Limits"=w309:T21, "Conditions"=w321:T25, "Overrides"=w296:T5, "Angular Limits"=w295:T6)
      n105 = Read from Binary File(5:w325, 11:w326) -> (2:w324:cluster{"x":dbl, "y":dbl, "th":dbl}[], 3:w314:refnum<file>)  [unwired: 4 in, 2 out]
      n106 = Read from Binary File(5:w322, 11:w314) -> (2:w298:cluster{"Time (s)":dbl, "Distance (ft)":dbl}, 3:w302:refnum<file>)  [unwired: 4 in, 2 out]
      n107 = Unbundle(w309) -> ("Velocity (fps)"=w307:dbl, "Accel (fps^2)"=w306:dbl, "Jerk (fps^3)"=w305:dbl, "StoopidFast (fps)"=w304:dbl)
      n108 = Bundle("Velocity (fps)"=w307, "Accel (fps^2)"=w306, "Jerk (fps^3)"=w305, "StoopidFast (fps)"=w304) -> (w308:T31)  [unwired: 1 in]
      n109 = Read from Binary File(5:FALSE, 11:w302) -> (2:w299:bool, 3:w301:refnum<file>)  [unwired: 4 in, 2 out]
    }
    frame "3.4" {
      # "Adding the zeroV overriede"
      n110 = Read from Binary File(5:T10 {"Robot Backwards"=FALSE, "Reverse Path"=FALSE} ("Cluster"), 11:w353) -> (2:w347:T10, 3:w350:refnum<file>)  [unwired: 4 in, 2 out]
      n111 = Read from Binary File(5:w360, 11:w350) -> (2:w357:T11, 3:w349:refnum<file>)  [unwired: 4 in, 2 out]
      n112 = Read from Binary File(5:w356, 11:w349) -> (0:w354:errorcluster, 2:w355:cluster{"Time (s)":dbl, T8, bool}[], 3:w348:refnum<file>)  [unwired: 4 in, 1 out]
      n113 = call "Convert Trajectory Data 4.0.vi"("pre 4.0"=w357) -> ("post 4.0"=w328:T1)
      n114 = Read from Binary File(5:T22 {"Sample Period (s)"=0.0, "Limits"={"Velocity (fps)"=0.0, "Accel (fps^2)"=0.0, "Jerk (fps^3)"=0.0, "StoopidFast (fps)"=0.0}, "Conditions"={"vInitial (fps)"=0.0, "vFinal (fps)"=0.0}, "Overrides"=[], "Angular Limits"={"Velocity (deg/s)"=0.0, "Accel (deg/s^2)"=0.0, "Jerk (deg/s^3)"=0.0}} ("output cluster"), 11:w348) -> (2:w364:T22, 3:w363:refnum<file>)  [unwired: 4 in, 2 out]
      n115 = Unbundle(w364) -> ("Sample Period (s)"=w340:dbl, "Limits"=w346:T21, "Conditions"=w358:T25, "Overrides"=w334:T5, "Angular Limits"=w333:T6)
      n116 = Read from Binary File(5:w362, 11:w363) -> (2:w361:cluster{"x":dbl, "y":dbl, "th":dbl}[], 3:w351:refnum<file>)  [unwired: 4 in, 2 out]
      n117 = Read from Binary File(5:w359, 11:w351) -> (2:w336:cluster{"Time (s)":dbl, "Distance (ft)":dbl}, 3:w339:refnum<file>)  [unwired: 4 in, 2 out]
      n118 = Unbundle(w346) -> ("Velocity (fps)"=w344:dbl, "Accel (fps^2)"=w343:dbl, "Jerk (fps^3)"=w342:dbl, "StoopidFast (fps)"=w341:dbl)
      n119 = Bundle("Velocity (fps)"=w344, "Accel (fps^2)"=w343, "Jerk (fps^3)"=w342, "StoopidFast (fps)"=w341) -> (w345:T31)  [unwired: 1 in]
      n120 = Read from Binary File(5:FALSE, 11:w339) -> (2:w337:bool, 3:w332:refnum<file>)  [unwired: 4 in, 2 out]
      n121 = Read from Binary File(5:cluster{"Drive Type":T3, "Path Type":T4} {"Drive Type"=enum."Nonholonomic", "Path Type"=enum."Clothoid"} ("Trajectory Meta"), 11:w332) -> (2:w329:cluster{"Drive Type":T3, "Path Type":T4}, 3:w330:refnum<file>)  [unwired: 4 in, 2 out]
    }
    frame "4.0" {
      # "Adding the zeroV overriede"
      n122 = Read from Binary File(5:T10 {"Robot Backwards"=FALSE, "Reverse Path"=FALSE} ("Cluster"), 11:w390) -> (2:w384:T10, 3:w387:refnum<file>)  [unwired: 4 in, 2 out]
      n123 = Read from Binary File(5:w365, 11:w387) -> (2:w394:T1, 3:w386:refnum<file>)  [unwired: 4 in, 2 out]
      n124 = Read from Binary File(5:w393, 11:w386) -> (0:w391:errorcluster, 2:w392:cluster{"Time (s)":dbl, T8, bool}[], 3:w385:refnum<file>)  [unwired: 4 in, 1 out]
      n125 = Read from Binary File(5:T22 {"Sample Period (s)"=0.0, "Limits"={"Velocity (fps)"=0.0, "Accel (fps^2)"=0.0, "Jerk (fps^3)"=0.0, "StoopidFast (fps)"=0.0}, "Conditions"={"vInitial (fps)"=0.0, "vFinal (fps)"=0.0}, "Overrides"=[], "Angular Limits"={"Velocity (deg/s)"=0.0, "Accel (deg/s^2)"=0.0, "Jerk (deg/s^3)"=0.0}} ("output cluster"), 11:w385) -> (2:w400:T22, 3:w399:refnum<file>)  [unwired: 4 in, 2 out]
      n126 = Unbundle(w400) -> ("Sample Period (s)"=w377:dbl, "Limits"=w383:T21, "Conditions"=w395:T25, "Overrides"=w371:T5, "Angular Limits"=w370:T6)
      n127 = Read from Binary File(5:w398, 11:w399) -> (2:w397:cluster{"x":dbl, "y":dbl, "th":dbl}[], 3:w388:refnum<file>)  [unwired: 4 in, 2 out]
      n128 = Read from Binary File(5:w396, 11:w388) -> (2:w373:cluster{"Time (s)":dbl, "Distance (ft)":dbl}, 3:w376:refnum<file>)  [unwired: 4 in, 2 out]
      n129 = Unbundle(w383) -> ("Velocity (fps)"=w381:dbl, "Accel (fps^2)"=w380:dbl, "Jerk (fps^3)"=w379:dbl, "StoopidFast (fps)"=w378:dbl)
      n130 = Bundle("Velocity (fps)"=w381, "Accel (fps^2)"=w380, "Jerk (fps^3)"=w379, "StoopidFast (fps)"=w378) -> (w382:T31)  [unwired: 1 in]
      n131 = Read from Binary File(5:FALSE, 11:w376) -> (2:w374:bool, 3:w369:refnum<file>)  [unwired: 4 in, 2 out]
      n132 = Read from Binary File(5:cluster{"Drive Type":T3, "Path Type":T4} {"Drive Type"=enum."Nonholonomic", "Path Type"=enum."Clothoid"} ("Trajectory Meta"), 11:w369) -> (2:w366:cluster{"Drive Type":T3, "Path Type":T4}, 3:w367:refnum<file>)  [unwired: 4 in, 2 out]
    }
    frame "4.2" {
      # "Adding the zeroV overriede"
      n133 = Read from Binary File(5:T10 {"Robot Backwards"=FALSE, "Reverse Path"=FALSE} ("Cluster"), 11:w429) -> (2:w423:T10, 3:w426:refnum<file>)  [unwired: 4 in, 2 out]
      n134 = Read from Binary File(5:w405, 11:w426) -> (2:w433:T1, 3:w425:refnum<file>)  [unwired: 4 in, 2 out]
      n135 = Read from Binary File(5:w432, 11:w425) -> (0:w430:errorcluster, 2:w431:cluster{"Time (s)":dbl, T8, bool}[], 3:w424:refnum<file>)  [unwired: 4 in, 1 out]
      n136 = Read from Binary File(5:T22 {"Sample Period (s)"=0.0, "Limits"={"Velocity (fps)"=0.0, "Accel (fps^2)"=0.0, "Jerk (fps^3)"=0.0, "StoopidFast (fps)"=0.0}, "Conditions"={"vInitial (fps)"=0.0, "vFinal (fps)"=0.0}, "Overrides"=[], "Angular Limits"={"Velocity (deg/s)"=0.0, "Accel (deg/s^2)"=0.0, "Jerk (deg/s^3)"=0.0}} ("output cluster"), 11:w424) -> (2:w439:T22, 3:w438:refnum<file>)  [unwired: 4 in, 2 out]
      n137 = Unbundle(w439) -> ("Sample Period (s)"=w416:dbl, "Limits"=w422:T21, "Conditions"=w434:T25, "Overrides"=w410:T5, "Angular Limits"=w409:T6)
      n138 = Read from Binary File(5:w437, 11:w438) -> (2:w436:cluster{"x":dbl, "y":dbl, "th":dbl}[], 3:w427:refnum<file>)  [unwired: 4 in, 2 out]
      n139 = Read from Binary File(5:w435, 11:w427) -> (2:w412:cluster{"Time (s)":dbl, "Distance (ft)":dbl}, 3:w415:refnum<file>)  [unwired: 4 in, 2 out]
      n140 = Unbundle(w422) -> ("Velocity (fps)"=w420:dbl, "Accel (fps^2)"=w419:dbl, "Jerk (fps^3)"=w418:dbl, "StoopidFast (fps)"=w417:dbl)
      n141 = Bundle("Velocity (fps)"=w420, "Accel (fps^2)"=w419, "Jerk (fps^3)"=w418, "StoopidFast (fps)"=w417) -> (w421:T31)  [unwired: 1 in]
      n142 = Read from Binary File(5:FALSE, 11:w415) -> (2:w413:bool, 3:w408:refnum<file>)  [unwired: 4 in, 2 out]
      n143 = Read from Binary File(5:cluster{"Drive Type":T3, "Path Type":T4} {"Drive Type"=enum."Nonholonomic", "Path Type"=enum."Clothoid"} ("Trajectory Meta"), 11:w408) -> (2:w406:cluster{"Drive Type":T3, "Path Type":T4}, 3:w404:refnum<file>)  [unwired: 4 in, 2 out]
      n144 = Read from Binary File(5:FALSE, 11:w404) -> (2:w401:bool, 3:w403:refnum<file>)  [unwired: 4 in, 2 out]
    }
  }
  "Zero V" <- w21
  "Reversals" <- w20
  "Commands out" <- w18
  "Points out" <- w16
  "Overall" <- w8
  "Trajectory Meta" <- w5
  "Trajectory Data" <- w2
  "Auto Align" <- w1
  n145 = Bundle("Sample Period (s)"=w23, w24, "Conditions"=w25, "Overrides"=w26, "Angular Limits"=w6) -> (→"Fields":T7)  [unwired: 1 in]
  n146 = Close File(refnum=w13) -> ()  [unwired: 1 in, 2 out]
